vi "Create Path.vi"(7 "Path Command":T1, 8 "error in (no error)":errorcluster) -> (0 "error out":errorcluster, 3 "created path":path)   [LabVIEW 2016, in "User Interface.lvlib"]
uses:
  User Interface.lvlib
  Create Path Command.ctl
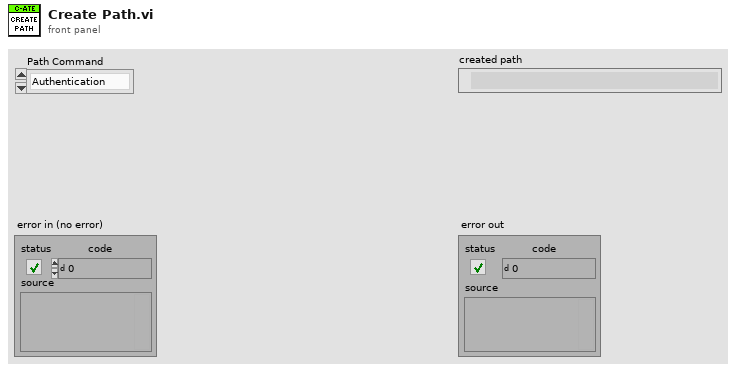
[diagram p1: front panel]
types:
  T1 = typedef "User Interface.lvlib/Create Path Command.ctl" = enum16{"Authentication", "Hardware", "Configuration", "Calibration", "Instrument", "Test Description", "Serial Data", "ARINC Data", "CAN Data", "Data", "Report", "Action log", "Error Log"}
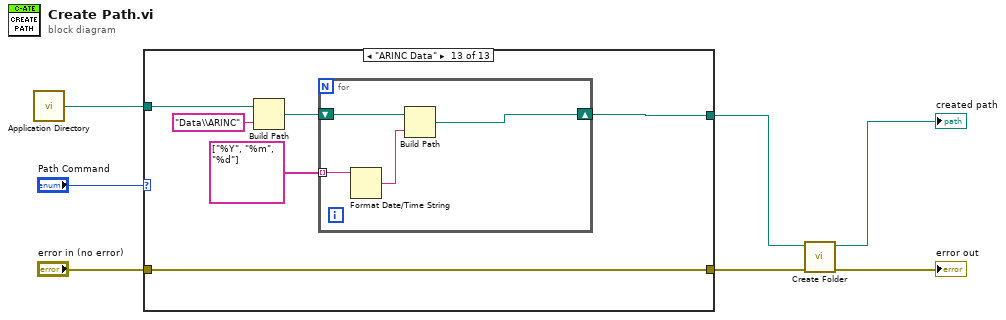
[diagram p0: block diagram]
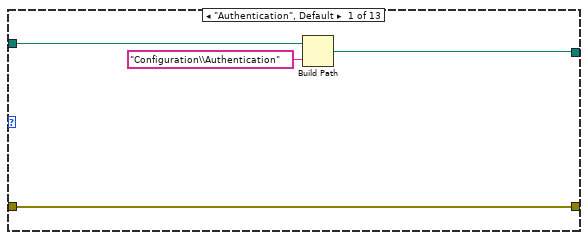
[diagram p2: hidden frame]
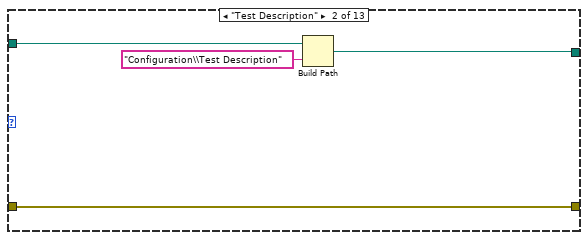
[diagram p3: hidden frame]
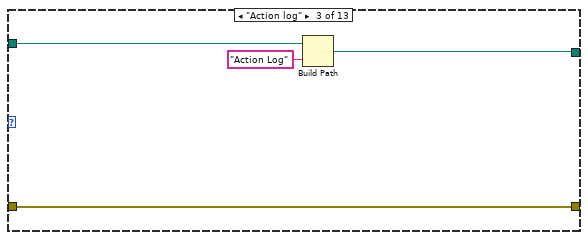
[diagram p4: hidden frame]
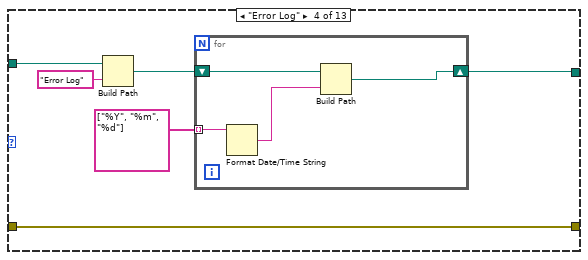
[diagram p5: hidden frame]
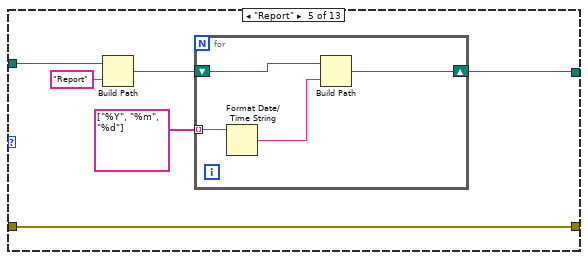
[diagram p6: hidden frame]
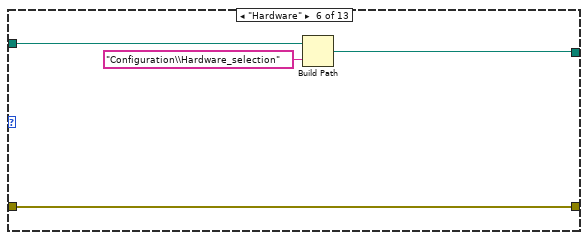
[diagram p7: hidden frame]
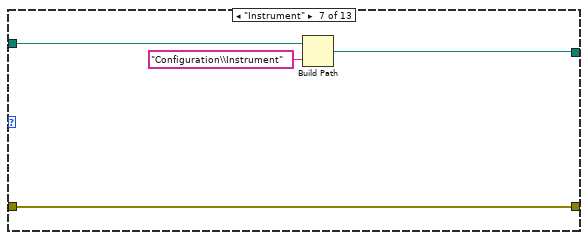
[diagram p8: hidden frame]
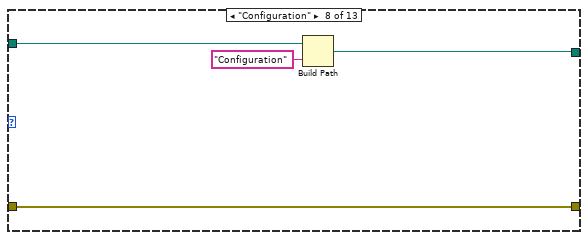
[diagram p9: hidden frame]
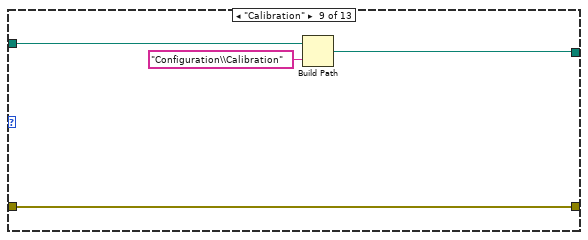
[diagram p10: hidden frame]
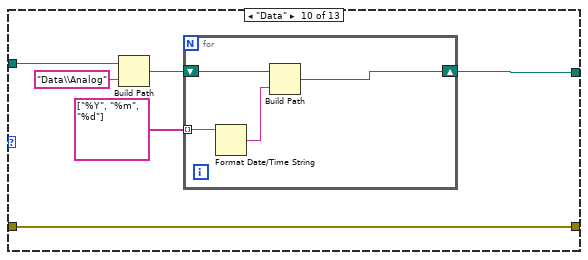
[diagram p11: hidden frame]
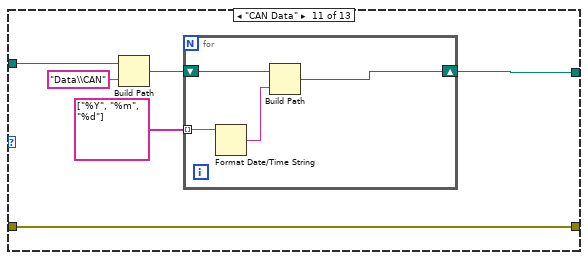
[diagram p12: hidden frame]
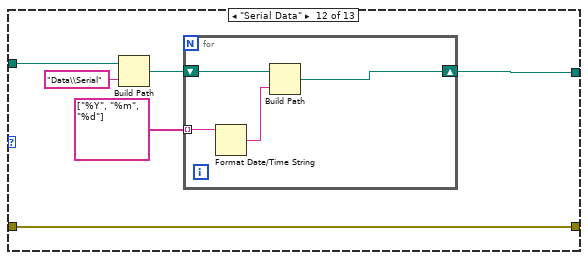
[diagram p13: hidden frame]
diagram:
  n1 = call <vilib>:"Application Directory.vi"() -> ("Application Directory"=w5:path)
  n2 = case shown="\"ARINC Data\"" "Path Command" {
    tunnel: "error in (no error)" -> [w8 w12 w16 w23 w33 w40 w44 w48 w52 w59 w69 w79 w89]
    tunnel: w5 -> [w11 w15 w19 w25 w35 w43 w47 w51 w55 w61 w71 w81 w91]
    tunnel: [w9 w13 w17 w20 w30 w41 w45 w49 w53 w56 w66 w76 w86] -> w3
    tunnel: [w8 w12 w16 w23 w33 w40 w44 w48 w52 w59 w69 w79 w89] -> w4
    frame "Authentication", Default {
      n3 = Build Path(base path=w11, name or relative path="Configuration\\Authentication") -> (appended path=w9:path)
    }
    frame "Test Description" {
      n4 = Build Path(base path=w15, name or relative path="Configuration\\Test Description") -> (appended path=w13:path)
    }
    frame "Action log" {
      n5 = Build Path(base path=w19, name or relative path="Action Log") -> (appended path=w17:path)
    }
    frame "Error Log" {
      n6 = Build Path(base path=w25, name or relative path="Error Log") -> (appended path=w21:path)
      n7 = for {
        tunnel: string[] ["%Y", "%m", "%d"] -> [w29] mode=indexing
        shift-right: [w26] -> w20
        shift-left: w21 -> [w28]
        n8 = Format Date/Time String(time format string (%c)=w29) -> (date/time string=w27:string)  [unwired: 2 in]
        n9 = Build Path(base path=w28, name or relative path=w27) -> (appended path=w26:path)
      }
    }
    frame "Report" {
      n10 = Build Path(base path=w35, name or relative path="Report") -> (appended path=w31:path)
      n11 = for {
        tunnel: string[] ["%Y", "%m", "%d"] -> [w39] mode=indexing
        shift-right: [w36] -> w30
        shift-left: w31 -> [w38]
        n12 = Format Date/Time String(time format string (%c)=w39) -> (date/time string=w37:string)  [unwired: 2 in]
        n13 = Build Path(base path=w38, name or relative path=w37) -> (appended path=w36:path)
      }
    }
    frame "Hardware" {
      n14 = Build Path(base path=w43, name or relative path="Configuration\\Hardware_selection") -> (appended path=w41:path)
    }
    frame "Instrument" {
      n15 = Build Path(base path=w47, name or relative path="Configuration\\Instrument") -> (appended path=w45:path)
    }
    frame "Configuration" {
      n16 = Build Path(base path=w51, name or relative path="Configuration") -> (appended path=w49:path)
    }
    frame "Calibration" {
      n17 = Build Path(base path=w55, name or relative path="Configuration\\Calibration") -> (appended path=w53:path)
    }
    frame "Data" {
      n18 = Build Path(base path=w61, name or relative path="Data\\Analog") -> (appended path=w58:path)
      n19 = for {
        tunnel: string[] ["%Y", "%m", "%d"] -> [w65] mode=indexing
        shift-right: [w62] -> w56
        shift-left: w58 -> [w64]
        n20 = Format Date/Time String(time format string (%c)=w65) -> (date/time string=w63:string)  [unwired: 2 in]
        n21 = Build Path(base path=w64, name or relative path=w63) -> (appended path=w62:path)
      }
    }
    frame "CAN Data" {
      n22 = Build Path(base path=w71, name or relative path="Data\\CAN") -> (appended path=w68:path)
      n23 = for {
        tunnel: string[] ["%Y", "%m", "%d"] -> [w75] mode=indexing
        shift-right: [w72] -> w66
        shift-left: w68 -> [w74]
        n24 = Format Date/Time String(time format string (%c)=w75) -> (date/time string=w73:string)  [unwired: 2 in]
        n25 = Build Path(base path=w74, name or relative path=w73) -> (appended path=w72:path)
      }
    }
    frame "Serial Data" {
      n26 = Build Path(base path=w81, name or relative path="Data\\Serial") -> (appended path=w78:path)
      n27 = for {
        tunnel: string[] ["%Y", "%m", "%d"] -> [w85] mode=indexing
        shift-right: [w82] -> w76
        shift-left: w78 -> [w84]
        n28 = Format Date/Time String(time format string (%c)=w85) -> (date/time string=w83:string)  [unwired: 2 in]
        n29 = Build Path(base path=w84, name or relative path=w83) -> (appended path=w82:path)
      }
    }
    frame "ARINC Data" {
      n30 = Build Path(base path=w91, name or relative path="Data\\ARINC") -> (appended path=w88:path)
      n31 = for {
        tunnel: string[] ["%Y", "%m", "%d"] -> [w95] mode=indexing
        shift-right: [w92] -> w86
        shift-left: w88 -> [w94]
        n32 = Format Date/Time String(time format string (%c)=w95) -> (date/time string=w93:string)  [unwired: 2 in]
        n33 = Build Path(base path=w94, name or relative path=w93) -> (appended path=w92:path)
      }
    }
  }
  n34 = call "Create Folder.vi"("error in (no error)"=w4, "Path"=w3) -> ("error out"=→"error out":errorcluster, "created path"=→"created path":path)  [unwired: 8 in]
